vi "Get Step Index By ID.vi"(8 "error in (no error)":errorcluster, 10 "ID":string, 11 "Project in":refnum<class "Project.lvclass">) -> (0 "error out":errorcluster, 2 "Index":i32, 3 "Project out":refnum<class "Project.lvclass">)   [LabVIEW 2015, in "Editor.lvclass"]
uses:
  Editor.lvclass
  Project.lvclass
  Step.lvclass
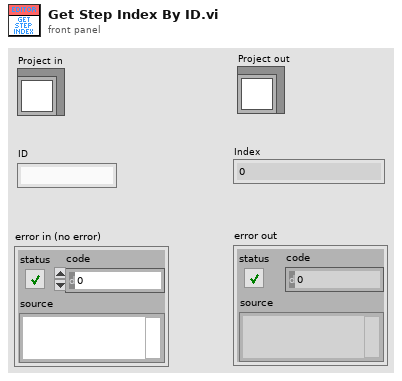
[diagram p1: front panel]
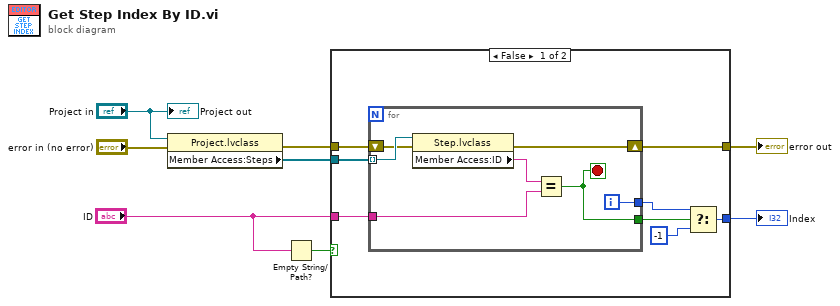
[diagram p0: block diagram]
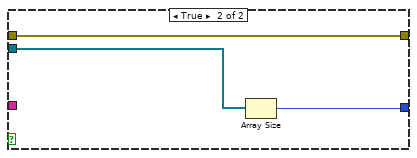
[diagram p2: hidden frame]
diagram:
  n1 = property class="Project.lvclass"(reference="Project in", error in="error in (no error)") -> (error out=w5:errorcluster, "Member Access:Steps"=w4:refnum<class "Step.lvclass">[])  [unwired: 1 out]
  n2 = Empty String/Path?(string/path="ID") -> (empty?=w2:bool)
  n3 = case shown="False" w2 {
    tunnel: "ID" -> [w16 _]
    tunnel: [w15 w26] -> w8
    tunnel: w5 -> [w14 w26]
    tunnel: w4 -> [w13 w25]
    tunnel: [w9 w24] -> w3
    frame False {
      n4 = for {
        shift-right: [w17] -> w15
        shift-left: w14 -> [w20]
        tunnel: w13 -> [w23] mode=indexing
        tunnel: w16 -> [w21]
        tunnel: [w19] -> w11
        tunnel: [w18] -> w12
        i -> [w19]
        stop <- w18 stop-if-true
        n5 = property class="Step.lvclass"(reference=w23, error in=w20) -> (error out=w17:errorcluster, "Member Access:ID"=w22:string)  [unwired: 1 out]
        n6 = Equal?(x=w22, y=w21) -> (x = y?=w18:bool)
      }
      n7 = Select(t=w11, s=w12, f=-1) -> (s? t:f=w9:i32)
    }
    frame True {
      n8 = Array Size(array=w25) -> (size(s)=w24:i32)
    }
  }
  "error out" <- w8
  "Index" <- w3
  "Project out" <- "Project in"
